vi "StreamProcess.Main.vi"(8 "error in (no error)":errorcluster, 9 "Refs":T1, 10 "FilterDVR.Ref":refnum<data-value>, 11 "Settings":T3) -> (0 "error out":errorcluster)   [LabVIEW 2025, in "bus_monitor_server_do.lvlib"]
uses:
  bus_monitor_server_do.lvlib
  Types/StreamProcess.State.ctl
  <resource>/objmgr/xnet.rc
  bus_monitor_server/RPC Messages/ni_bus_monitor_api_Frame.ctl
  bus_monitor_server/bus_monitor_server.lvlib
  bus_monitor_server/RPC Service/Bus_Monitor_API/Bus_Monitor_API.lvclass
  bus_monitor_server/RPC Messages/ni_bus_monitor_api_StreamBusReply.ctl
  <vilib>/xnet/xnet.llb/XNET Create Session (Frame Input Stream).vi
  <vilib>/xnet/xnet.llb/XNET Read (State CAN Comm).vi
  <vilib>/xnet/xnet.llb/XNET Read (Frame CAN).vi
  bus_monitor_server/RPC Messages/ni_bus_monitor_api_ErrorInfo.ctl
  bus_monitor_server/RPC Messages/ni_bus_monitor_api_LastCommError.ctl
  bus_monitor_server/RPC Messages/ni_bus_monitor_api_CommState.ctl
  bus_monitor_server/RPC Messages/ni_bus_monitor_api_CanCommState.ctl
  <vilib>/xnet/xnet.llb/XNET CAN Comm State.ctl
  <vilib>/xnet/xnet.llb/XNET CAN Last Err.ctl
  <vilib>/xnet/xnet.llb/XNET CAN Comm.ctl
  <vilib>/xnet/xnet.llb/XNET Frame Type CAN.ctl
  <vilib>/xnet/xnet.llb/XNET Frame CAN.ctl
  Types/XNET.InitialSettings.ctl
  <vilib>/gRPC/LabVIEW gRPC Library/Shared/grpcId.ctl
  <vilib>/gRPC/LabVIEW gRPC Library/grpc-lvsupport-release.lvlib
  Types/StreamProcess.InputRefs.ctl
  bus_monitor_server/RPC Messages/ni_bus_monitor_api_FrameFilter.ctl
  bus_monitor_server/RPC Messages/ni_bus_monitor_api_DirectionFilter.ctl
  bus_monitor_server/RPC Messages/ni_bus_monitor_api_FilterInfo.ctl
  bus_monitor_server/RPC Messages/ni_bus_monitor_api_FdIsoMode.ctl
  bus_monitor_server/RPC Messages/ni_bus_monitor_api_Termination.ctl
  bus_monitor_server/RPC Messages/ni_bus_monitor_api_CanMode.ctl
  bus_monitor_server/RPC Messages/ni_bus_monitor_api_ConnectSettings.ctl
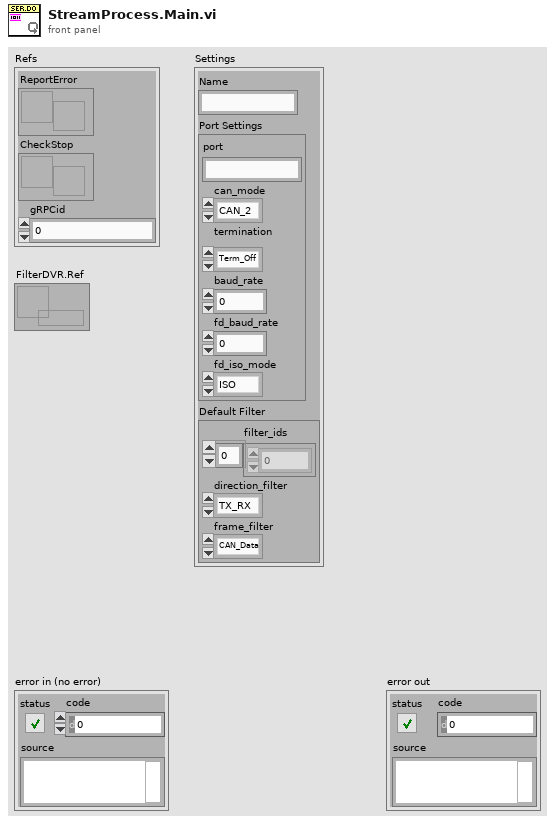
[diagram p1: front panel]
types:
  T1 = typedef "bus_monitor_server_do.lvlib/StreamProcess.InputRefs.ctl" = cluster{"ReportError":refnum<notifier>, "CheckStop":refnum<notifier>, "gRPCid":T2}
  T2 = typedef "grpc-lvsupport-release.lvlib/grpcId.ctl" = u64
  T3 = typedef "bus_monitor_server_do.lvlib/XNET.InitialSettings.ctl" = cluster{"Name":string, "Port Settings":T4, "Default Filter":T8}
  T4 = typedef "bus_monitor_server.lvlib/ni_bus_monitor_api_ConnectSettings.ctl" = cluster{"port":string, "can_mode":T5, "termination":T6, "baud_rate":u64, "fd_baud_rate":u64, "fd_iso_mode":T7}
  T5 = typedef "bus_monitor_server.lvlib/ni_bus_monitor_api_CanMode.ctl" = enum32{"CAN_2", "CAN_FD", "CAN_FD_BRS"}
  T6 = typedef "bus_monitor_server.lvlib/ni_bus_monitor_api_Termination.ctl" = enum32{"Term_Off", "Term_On"}
  T7 = typedef "bus_monitor_server.lvlib/ni_bus_monitor_api_FdIsoMode.ctl" = enum32{"ISO", "Non_ISO", "ISO_Legacy"}
  T8 = typedef "bus_monitor_server.lvlib/ni_bus_monitor_api_FilterInfo.ctl" = cluster{"filter_ids":u32[], "direction_filter":T9, "frame_filter":T10}
  T9 = typedef "bus_monitor_server.lvlib/ni_bus_monitor_api_DirectionFilter.ctl" = enum32{"TX_RX", "RX", "TX"}
  T10 = typedef "bus_monitor_server.lvlib/ni_bus_monitor_api_FrameFilter.ctl" = enum32{"CAN_Data", "CAN_Remote", "CAN_Bus_Error", "CAN_2_Data", "CAN_FD_Data", "CAN_FD_BRS_Data", "J1939_Data", "Delay", "Log_Trigger", "Start_Trigger", "All"}
  T11 = typedef "bus_monitor_server_do.lvlib/StreamProcess.State.ctl" = enum8{"Open XNET Session", "Publish", "Cleanup"}
  T12 = typedef "bus_monitor_server.lvlib/ni_bus_monitor_api_StreamBusReply.ctl" = cluster{"can_comm_state":T13, "frame":T16[], "error":T17}
  T13 = typedef "bus_monitor_server.lvlib/ni_bus_monitor_api_CanCommState.ctl" = cluster{"fault_code":i32, "fault":bool, "comm_state":T14, "last_comm_error":T15, "receive_error_counter":u32, "transmit_error_counter":u32, "transceiver_error":bool, "sleep":bool}
  T14 = typedef "bus_monitor_server.lvlib/ni_bus_monitor_api_CommState.ctl" = enum32{"Error_Active", "Error_Passive", "Bus_Off", "Init"}
  T15 = typedef "bus_monitor_server.lvlib/ni_bus_monitor_api_LastCommError.ctl" = enum32{"None", "Stuff", "Form", "ACK", "Bit1", "Bit0", "CRC"}
  T16 = typedef "bus_monitor_server.lvlib/ni_bus_monitor_api_Frame.ctl" = cluster{"timestamp":dbl, "payload":u8[], "identifier":u32, "frame_type":u32, "extended":bool, "echo":bool}
  T17 = typedef "bus_monitor_server.lvlib/ni_bus_monitor_api_ErrorInfo.ctl" = errorcluster
  T18 = typedef "XNET Frame CAN.ctl" = cluster{"timestamp":timestamp, "payload":u8[], "identifier":u32, "type":T19, "extended?":bool, "echo?":bool}
  T19 = typedef "XNET Frame Type CAN.ctl" = u8
  T20 = typedef "XNET CAN Comm.ctl" = cluster{"fault code":i32, "fault?":bool, "communication state":T21, "last error":T22, "receive error counter":u8, "transmit error counter":u8, "transceiver error?":bool, "sleep?":bool}
  T21 = typedef "XNET CAN Comm State.ctl" = u8
  T22 = typedef "XNET CAN Last Err.ctl" = u8
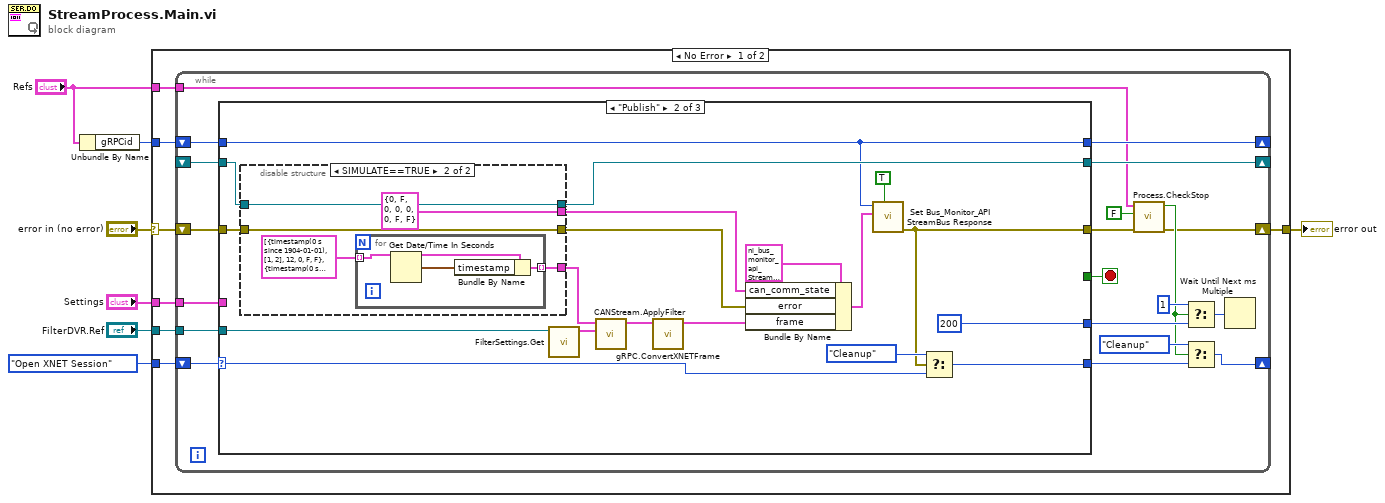
[diagram p0: block diagram]
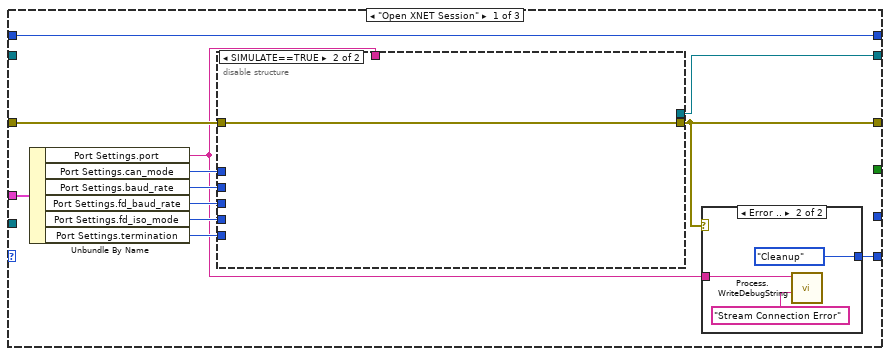
[diagram p2: hidden frame]
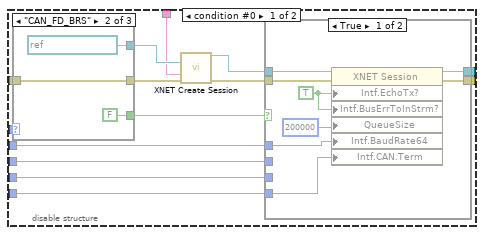
[diagram p3: hidden frame]
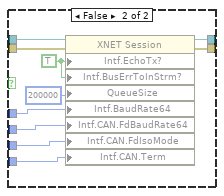
[diagram p4: hidden frame]
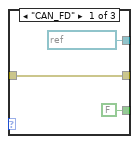
[diagram p5: hidden frame]
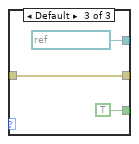
[diagram p6: hidden frame]
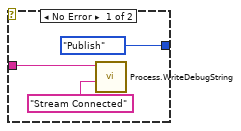
[diagram p7: hidden frame]
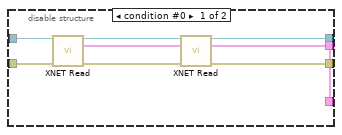
[diagram p8: hidden frame]
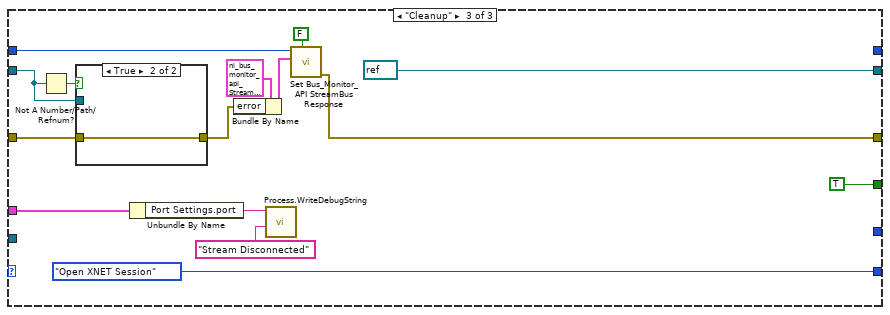
[diagram p9: hidden frame]
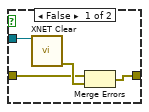
[diagram p10: hidden frame]
diagram:
  n1 = Unbundle By Name("Refs") -> ("gRPCid"=w1:T2)
  n2 = case shown="No Error" "error in (no error)" {
    selector: "error in (no error)" -> [w9 w150]
    tunnel: [w14 w150] -> w7
    tunnel: StreamProcess.State."Open XNET Session" -> [w13 _]
    tunnel: "Settings" -> [w12 _]
    tunnel: "Refs" -> [w11 _]
    tunnel: w1 -> [w10 _]
    tunnel: "FilterDVR.Ref" -> [w8 _]
    frame No Error {
      n3 = while {
        shift-right: [w24] -> _
        shift-left: w13 -> [w34]
        shift-right: [w33] -> _
        shift-left: w10 -> [w32]
        shift-right: [w16] -> w14
        shift-left: w9 -> [w31]
        shift-right: [w29] -> _
        shift-left: _ -> [w28]
        tunnel: w12 -> [w25]
        tunnel: w11 -> [w18]
        tunnel: w8 -> [w15]
        stop <- w30 stop-if-true
        n4 = case shown="\"Publish\"" w34 {
          selector: w34 -> [_ w113 _]
          tunnel: [w35 w112 StreamProcess.State."Open XNET Session"] -> w26
          tunnel: [w46 w101 _] -> w33
          tunnel: w32 -> [w46 w101 w135]
          tunnel: [w44 w100 w131] -> w17
          tunnel: w31 -> [w39 w108 w140]
          tunnel: [_ _ TRUE] -> w30
          tunnel: [w45 w107 refnum<k21> refnum ("session out")] -> w29
          tunnel: w28 -> [_ w110 w142]
          tunnel: [_ u32 200 ("millisecond multiple") _] -> w23
          tunnel: w25 -> [w43 _ w139]
          tunnel: w15 -> [_ w95 _]
          frame "Open XNET Session" {
            n5 = Unbundle By Name(w43) -> ("Port Settings.port"=w36:string, "Port Settings.can_mode"=w40:T5, "Port Settings.baud_rate"=w38:u64, "Port Settings.fd_baud_rate"=w37:u64, "Port Settings.fd_iso_mode"=w41:T7, "Port Settings.termination"=w42:T6)
            n6 = disable-structure shown="SIMULATE==TRUE" {
              disable-tunnel: [w59 _] -> w45
              disable-tunnel: [w57 w88] -> w44
              disable-tunnel: w42 -> [w56 _]
              disable-tunnel: w41 -> [w52 _]
              disable-tunnel: w40 -> [w51 _]
              disable-tunnel: w39 -> [w50 w88]
              disable-tunnel: w38 -> [w49 _]
              disable-tunnel: w37 -> [w48 _]
              disable-tunnel: w36 -> [w47 _]
              frame condition #0 {
                n7 = case shown="\"CAN_FD_BRS\"" w51 {
                  tunnel: [refnum<k21> ":can_fd:" ("cluster (:memory:)") refnum<k21> ":can_fd_brs:" ("cluster (:memory:)") refnum<k21> ":memory:" ("cluster (:memory:)")] -> w55
                  tunnel: w50 -> [w79 w82 w85]
                  tunnel: [w79 w82 w85] -> w54
                  tunnel: [FALSE FALSE TRUE] -> w53
                  frame "CAN_FD" {
                  }
                  frame "CAN_FD_BRS" {
                  }
                  frame Default {
                  }
                }
                n8 = call-poly <vilib>:"XNET Create Session.vi"("cluster (:memory:)"=w55, "interface"=w47, "error in (no error)"=w54) -> ("session out"=w60:refnum<k21>, "error out"=w58:errorcluster)  [unwired: 11 out]
                n9 = case shown="True" w53 {
                  tunnel: w60 -> [w68 w78]
                  tunnel: [w67 w77] -> w59
                  tunnel: w58 -> [w66 w76]
                  tunnel: [w65 w75] -> w57
                  tunnel: w56 -> [w62 w72]
                  tunnel: w49 -> [w61 w71]
                  tunnel: w52 -> [_ w70]
                  tunnel: w48 -> [_ w69]
                  frame True {
                    w63 = TRUE ("Interface:Echo Transmit?")
                    n10 = property class="XNET Session"(reference=w68, error in=w66, "Intf.EchoTx?"=w63, "Intf.BusErrToInStrm?"=w63, "QueueSize"=u32 200000 ("Queue Size"), "Intf.BaudRate64"=w61, "Intf.CAN.Term"=w62) -> (reference out=w67:refnum<k21>, error out=w65:errorcluster)
                  }
                  frame False {
                    w73 = TRUE ("Interface:Echo Transmit?")
                    n11 = property class="XNET Session"(reference=w78, error in=w76, "Intf.EchoTx?"=w73, "Intf.BusErrToInStrm?"=w73, "QueueSize"=u32 200000 ("Queue Size"), "Intf.BaudRate64"=w71, "Intf.CAN.FdBaudRate64"=w69, "Intf.CAN.FdIsoMode"=w70, "Intf.CAN.Term"=w72) -> (reference out=w77:refnum<k21>, error out=w75:errorcluster)
                  }
                }
              }
              frame condition #1 (active) {
              }
            }
            n12 = case shown="Error .." w44 {
              tunnel: w36 -> [w90 w93]
              tunnel: [StreamProcess.State."Publish" StreamProcess.State."Cleanup"] -> w35
              frame No Error {
                n13 = call "Process.WriteDebugString.vi"("State"="Stream Connected", "Name"=w90) -> ()  [unwired: 9 in, 1 out]
              }
              frame Error {
                n14 = call "Process.WriteDebugString.vi"("State"="Stream Connection Error", "Name"=w93) -> ()  [unwired: 9 in, 1 out]
              }
            }
          }
          frame "Publish" {
            n15 = disable-structure shown="SIMULATE==TRUE" {
              disable-tunnel: w110 -> [w121 w125]
              disable-tunnel: w108 -> [w120 w126]
              disable-tunnel: [w117 w125] -> w107
              disable-tunnel: [w116 T20 {"fault code"=0, "fault?"=FALSE, "communication state"=0, "last error"=0, "receive error counter"=0, "transmit error counter"=0, "transceiver error?"=FALSE, "sleep?"=FALSE} ("CAN comm")] -> w106
              disable-tunnel: [w115 w122] -> w105
              disable-tunnel: [w114 w126] -> w96
              frame condition #0 {
                n16 = call-poly <vilib>:"XNET Read.vi"("session in"=w121, "error in (no error)"=w120) -> ("session out"=w118:refnum<k21>, "data"=w115:T18[], "error out"=w119:errorcluster)  [unwired: 11 out]
                n17 = call-poly <vilib>:"XNET Read.vi"("session in"=w118, "error in (no error)"=w119) -> ("session out"=w117:refnum<k21>, "CAN comm"=w116:T20, "error out"=w114:errorcluster)  [unwired: 11 out]
              }
              frame condition #1 (active) {
                n18 = for {
                  tunnel: T18[] [{"timestamp"=timestamp(0 s since 1904-01-01), "payload"=[1, 2], "identifier"=12, "type"=0, "extended?"=FALSE, "echo?"=FALSE}, {"timestamp"=timestamp(0 s since 1904-01-01), "payload"=[3, 4], "identifier"=13, "type"=0, "extended?"=FALSE, "echo?"=FALSE}] ("frames in") -> [w129] mode=indexing
                  tunnel: [w128] -> w122 mode=indexing
                  n19 = Get Date/Time In Seconds() -> (seconds since 1Jan1904=w127:timestamp)
                  n20 = Bundle By Name(cluster=w129, "timestamp"=w127) -> (w128:T18)
                }
              }
            }
            n21 = call "FilterSettings.Get.vi"("FilterDVR.Ref"=w95) -> ("Filter"=w104:T8)  [unwired: 9 in, 1 out]
            n22 = call "CANStream.ApplyFilter.vi"("Filter"=w104, "frames in"=w105) -> ("frames out"=w103:T18[])  [unwired: 9 in]
            n23 = call "gRPC.ConvertXNETFrame.vi"("frames in"=w103) -> ("Array"=w102:T16[])  [unwired: 10 in]
            n24 = Bundle By Name(cluster=T12 {"can_comm_state"={"fault_code"=0, "fault"=FALSE, "comm_state"=enum."Error_Active", "last_comm_error"=enum."None", "receive_error_counter"=0, "transmit_error_counter"=0, "transceiver_error"=FALSE, "sleep"=FALSE}, "frame"=[], "error"={"status"=FALSE, "code"=0, "source"=""}} ("Message Data"), "can_comm_state"=w106, "error"=w96, "frame"=w102) -> (w99:T12)
            n25 = call "Set Bus_Monitor_API StreamBus Response.vi"("Streaming? (F)"=TRUE, "Message Data"=w99, "gRPCid in"=w101) -> ("error out"=w100:errorcluster)  [unwired: 8 in]
            n26 = Select(t=StreamProcess.State."Cleanup", s=w100, f=w113) -> (s? t:f=w112:T11)
          }
          frame "Cleanup" {
            n27 = Not A Number/Path/Refnum?(number/path/refnum=w142) -> (NaN/Path/Refnum?=w141:bool)
            n28 = case shown="True" w141 {
              tunnel: w140 -> [w145 w149]
              tunnel: [w146 w149] -> w132
              tunnel: w142 -> [w148 _]
              frame False {
                n29 = call <vilib>:"XNET Clear.vi"("session in"=w148) -> ("error out"=w147:errorcluster)  [unwired: 14 in]
                n30 = Merge Errors(w145, w147) -> (w146:errorcluster)
              }
              frame True {
              }
            }
            n31 = Unbundle By Name(w139) -> ("Port Settings.port"=w138:string)
            n32 = Bundle By Name(cluster=T12 {"can_comm_state"={"fault_code"=0, "fault"=FALSE, "comm_state"=enum."Error_Active", "last_comm_error"=enum."None", "receive_error_counter"=0, "transmit_error_counter"=0, "transceiver_error"=FALSE, "sleep"=FALSE}, "frame"=[], "error"={"status"=FALSE, "code"=0, "source"=""}} ("Message Data"), "error"=w132) -> (w133:T12)
            n33 = call "Process.WriteDebugString.vi"("State"="Stream Disconnected", "Name"=w138) -> ()  [unwired: 9 in, 1 out]
            n34 = call "Set Bus_Monitor_API StreamBus Response.vi"("Streaming? (F)"=FALSE, "Message Data"=w133, "gRPCid in"=w135) -> ("error out"=w131:errorcluster)  [unwired: 8 in]
          }
        }
        n35 = call "Process.CheckStop.vi"("error in (no error)"=w17, "Stop Async on Error?"=FALSE, "LocalInterface.Refs"=w18) -> ("error out"=w16:errorcluster, "Stop"=w20:bool)  [unwired: 7 in]
        n36 = Select(t=u32 1, s=w20, f=w23) -> (s? t:f=w22:u32)
        n37 = Select(t=StreamProcess.State."Cleanup" ("y"), s=w20, f=w26) -> (s? t:f=w24:T11)
        n38 = Wait Until Next ms Multiple(millisecond multiple=w22) -> ()  [unwired: 1 out]
      }
    }
    frame Error {
    }
  }
  "error out" <- w7
